vi "X_Y_Read.vi"(8 "error in (no error)":errorcluster, 10 "Address to Read":string="68", 11 "VISA resource name In":refnum<visa-resource-name>) -> (0 "error out":errorcluster, 2 "Number Out":u32, 3 "VISA resource name out":refnum<visa-resource-name>)   [LabVIEW 2017]
uses:
  <vilib>/Instr/_visa.llb/Select Event Type.ctl
panel:
  out "concatenated string":string
  out "Lower Byte":string
  out "Upper Byte":string
  out "First Response":string
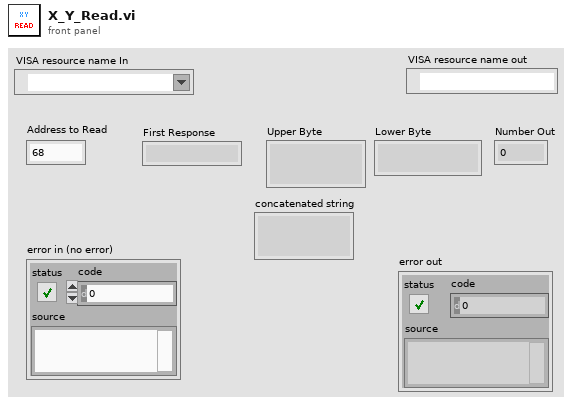
[diagram p1: front panel]
types:
  T1 = typedef "Select Event Type.ctl" = u32
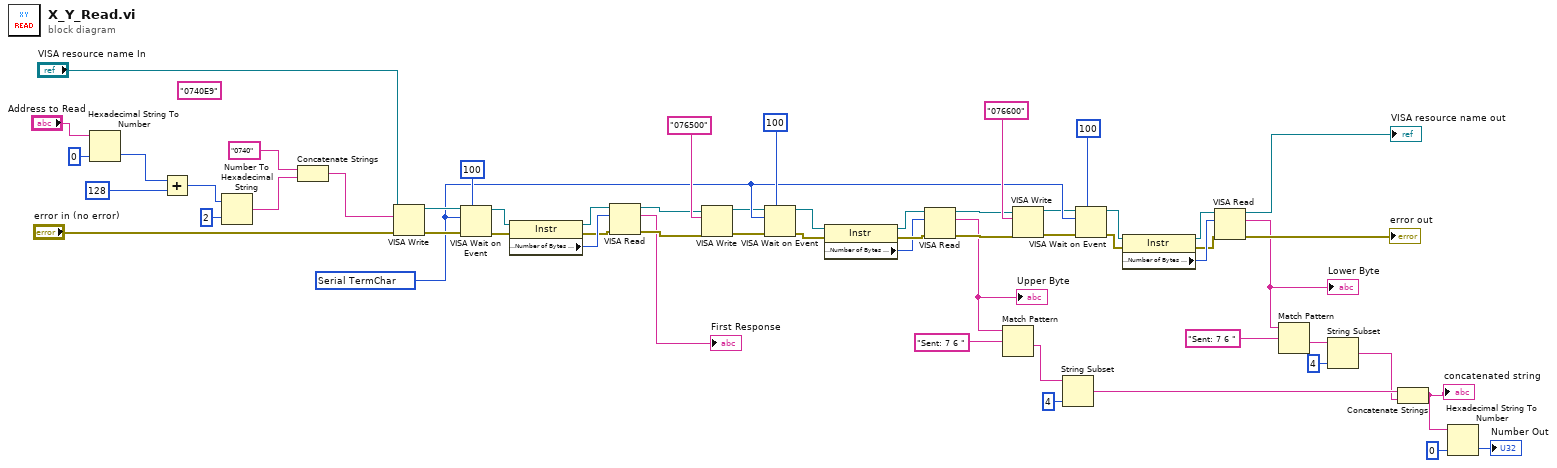
[diagram p0: block diagram]
diagram:
  w33 = T1 1073684516 items=["Service Request"=1073684491, "Trigger"=3221168138, "Clear"=1073684493, "VXI Signal"=1073684512, "VXI/VME Interrupt"=3221168161, "VXI/VME Sysfail"=1073684509, "VXI/VME Sysreset"=1073684510, "GPIB CIC"=1073684498, "GPIB Talk"=1073684499, "GPIB Listen"=1073684500, "PXI Interrupt"=1073684514, "Serial Break"=1073684515, "Serial TermChar"=1073684516, "Serial CTS"=1073684521, "Serial DSR"=1073684522, "Serial DCD"=1073684524, "Serial RI"=1073684526, "Serial Character"=1073684533, "USB Interrupt"=1073684535, "All Enabled"=1073709055] ("Event Type")
  (unwired) "0740E9" ("write buffer")
  n1 = Hexadecimal String To Number(string="Address to Read", default (0uL)=u32 0 ("default (0 U32)")) -> (number=w22:u32)  [unwired: 1 in, 1 out]
  n2 = Add(x=w22, y=u32 128) -> (x+y=w43:u32)
  n3 = Number To Hexadecimal String(1:i16 2 ("width (-)"), 2:w43) -> (0:w41:string)
  n4 = Concatenate Strings("0740" ("write buffer"), w41) -> (w40:string)
  n5 = VISA Write(VISA resource name="VISA resource name In", write buffer=w40, error in (no error)="error in (no error)") -> (VISA resource name out=w56:refnum<visa-resource-name>, error out=w57:errorcluster)  [unwired: 1 out]
  n6 = VISA Wait on Event(7:u32 100 ("timeout (0)"), 8:w57, 10:w33, 11:w56) -> (0:w53:errorcluster, 3:w54:refnum<visa-resource-name>)  [unwired: 1 in, 2 out]
  n7 = property class="Instr"(reference=w54, error in=w53) -> (reference out=w50:refnum<visa-resource-name>, error out=w51:errorcluster, "Serial Settings:Number of Bytes at Serial Port"=w52:u32)
  n8 = VISA Read(VISA resource name=w50, byte count=w52, error in (no error)=w51) -> (VISA resource name out=w48:refnum<visa-resource-name>, read buffer=→"First Response":string, error out=w49:errorcluster)  [unwired: 1 out]
  n9 = VISA Write(VISA resource name=w48, write buffer="076500", error in (no error)=w49) -> (VISA resource name out=w13:refnum<visa-resource-name>, error out=w14:errorcluster)  [unwired: 1 out]
  n10 = VISA Wait on Event(7:u32 100 ("timeout (0)"), 8:w14, 10:w33, 11:w13) -> (0:w8:errorcluster, 3:w9:refnum<visa-resource-name>)  [unwired: 1 in, 2 out]
  n11 = property class="Instr"(reference=w9, error in=w8) -> (reference out=w12:refnum<visa-resource-name>, error out=w11:errorcluster, "Serial Settings:Number of Bytes at Serial Port"=w10:u32)
  n12 = VISA Read(VISA resource name=w12, byte count=w10, error in (no error)=w11) -> (VISA resource name out=w34:refnum<visa-resource-name>, read buffer=w29:string, error out=w35:errorcluster)  [unwired: 1 out]
  "Upper Byte" <- w29
  n13 = Match Pattern(string=w29, regular expression="Sent: 7 6 ") -> (after substring=w19:string)  [unwired: 1 in, 3 out]
  n14 = VISA Write(VISA resource name=w34, write buffer="076600", error in (no error)=w35) -> (VISA resource name out=w2:refnum<visa-resource-name>, error out=w1:errorcluster)  [unwired: 1 out]
  n15 = String Subset(string=w19, length (rest)=4 ("length (rest)")) -> (substring=w20:string)  [unwired: 1 in]
  n16 = VISA Wait on Event(7:u32 100 ("timeout (0)"), 8:w1, 10:w33, 11:w2) -> (0:w7:errorcluster, 3:w6:refnum<visa-resource-name>)  [unwired: 1 in, 2 out]
  n17 = property class="Instr"(reference=w6, error in=w7) -> (reference out=w3:refnum<visa-resource-name>, error out=w4:errorcluster, "Serial Settings:Number of Bytes at Serial Port"=w5:u32)
  n18 = VISA Read(VISA resource name=w3, byte count=w5, error in (no error)=w4) -> (VISA resource name out=→"VISA resource name out":refnum<visa-resource-name>, read buffer=w26:string, error out=→"error out":errorcluster)  [unwired: 1 out]
  "Lower Byte" <- w26
  n19 = Match Pattern(string=w26, regular expression="Sent: 7 6 ") -> (after substring=w16:string)  [unwired: 1 in, 3 out]
  n20 = String Subset(string=w16, length (rest)=4 ("length (rest)")) -> (substring=w15:string)  [unwired: 1 in]
  n21 = Concatenate Strings(w20, w15) -> (w25:string)
  "concatenated string" <- w25
  n22 = Hexadecimal String To Number(string=w25, default (0uL)=u32 0 ("default (0 U32)")) -> (number=→"Number Out":u32)  [unwired: 1 in, 1 out]
